vi "synchronization .vi"(0 "appended path":path, 5 "prb_num":dbl, 7 "rbstart":dbl, 9 "rxData":cdb[](array[numeric]), 11 "error in (no error)":errorcluster caption="错误输入（无错误）", 12 "UL_subframe_num":dbl, 13 "cellid":dbl) -> (1 "rxmodify":cdb[](array[numeric]), 4 "timestart,":dbl, 6 "corrdata":dbl[](array[numeric]), 14 "error IO":errorcluster)   [LabVIEW 2015]
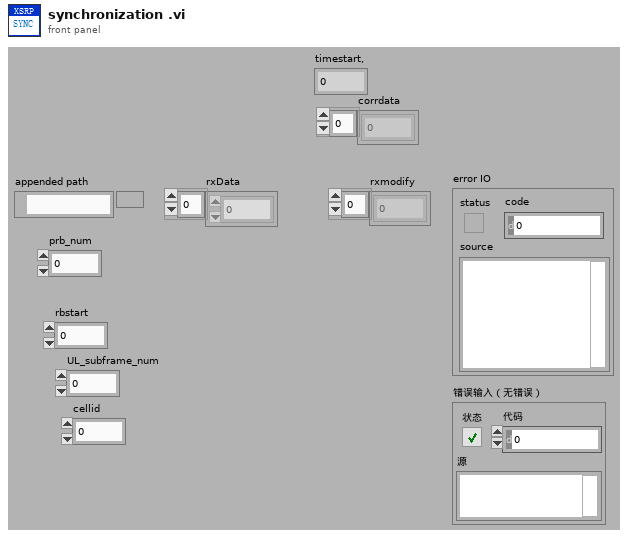
[diagram p1: front panel]
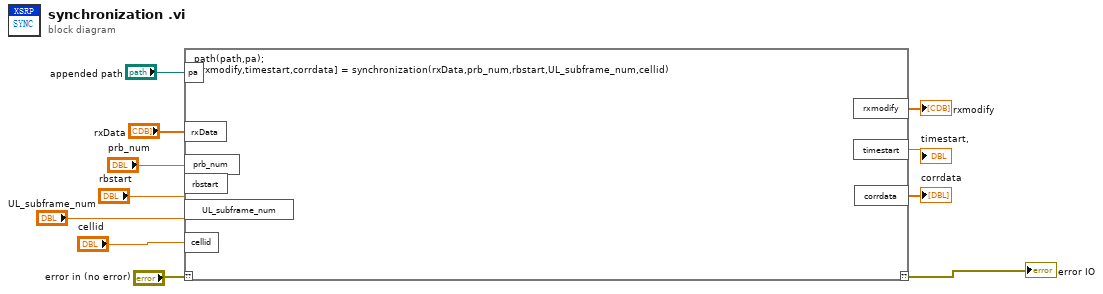
[diagram p0: block diagram]
diagram:
  n1 = script code="path(path,pa);\n[ rxmodify,timestart,corrdata] = synchronization(rxData,prb_num,rbstart,UL_subframe_num,cellid)"("??"="error in (no error)", "pa"="appended path", "rxData"="rxData", "prb_num"="prb_num", "rbstart"="rbstart", "UL_subframe_num"="UL_subframe_num", "cellid"="cellid") -> ("??"=→"error IO":errorcluster, "rxmodify"=→"rxmodify":cdb[], "timestart"=→"timestart,":dbl, "corrdata"=→"corrdata":dbl[])
